vi "GEA3 EMV Manual Mode.vi"(8 "error in (no error)":errorcluster, 10 "Manual Mode?":bool, 11 ".NET Refnum in":refnum<k24>) -> (0 "error out":errorcluster, 3 "GEA2 Reference Out":refnum<k24>)   [LabVIEW 2019]
uses:
  C:/TechnologyLab/NI-2010/Drivers/GEA3 Toolkit/GEA3 DLL Source/GeaCommunication.dll
  GEA3 DLL Source/GeaCommunication.dll
  type defs/ERD Write Data In.ctl
  type defs/Data Type.ctl
  library/GEA2_Toolkit.lvlib
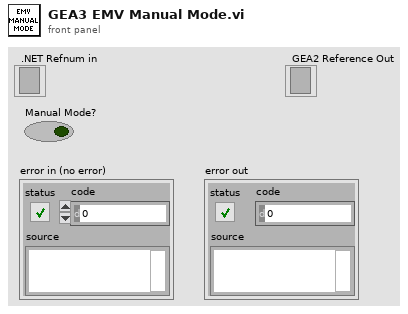
[diagram p1: front panel]
types:
  T1 = typedef "GEA2_Toolkit.lvlib/ERD Write Data In.ctl" = cluster{"ERD Number":u16, "Data Type":T2, "Data":string}
  T2 = typedef "GEA2_Toolkit.lvlib/Data Type.ctl" = enum16{"string", "boolean", "uint8_t", "uint16_t", "uint32_t", "uint64_t", "int8_t", "int16_t", "int32_t", "int64_t"}
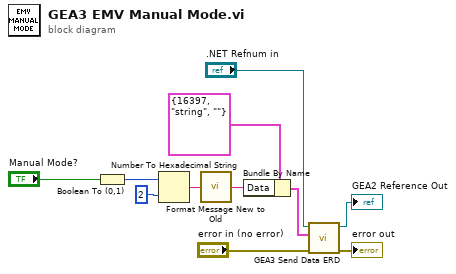
[diagram p0: block diagram]
diagram:
  n1 = Boolean To (0,1)(Boolean="Manual Mode?") -> (0, 1=w7:i16)
  n2 = Number To Hexadecimal String(1:i16 2 ("width (-)"), 2:w7) -> (0:w8:string)
  n3 = call "Format Message New to Old.vi"("Raw Message In"=w8) -> ("Conv Message Out"=w10:string)  [unwired: 14 in]
  n4 = Bundle By Name(cluster=T1 {"ERD Number"=16397, "Data Type"=enum."string", "Data"=""} ("ERD Write Data In"), "Data"=w10) -> (w5:T1)
  n5 = call "GEA3 Send Data ERD.vi"("error in (no error)"="error in (no error)", "ERD Write Data In"=w5, ".NET Refnum in"=".NET Refnum in") -> ("error out"=→"error out":errorcluster, "GEA2 Reference Out"=→"GEA2 Reference Out":refnum<k24>)  [unwired: 5 in, 2 out]
